vi "Json Parse.vi"(8 "error in (no error)":errorcluster, 11 "JSON":string) -> (0 "error out":errorcluster, 3 "variant":variant)   [LabVIEW 2020, in "WebView2 Control.xctl"]
uses:
  WebView2 Control.xctl
  System.Web.Extensions
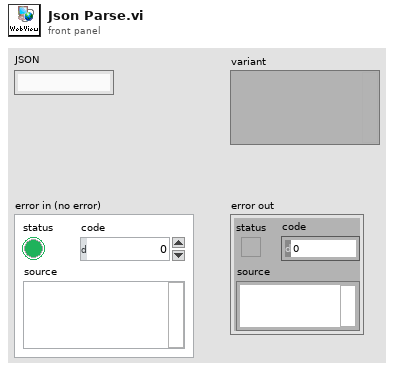
[diagram p1: front panel]
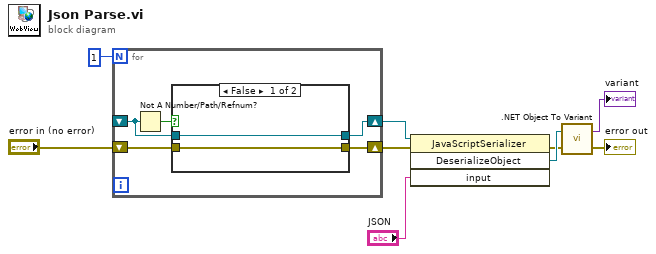
[diagram p0: block diagram]
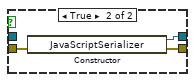
[diagram p2: hidden frame]
diagram:
  n1 = for {
    N: 1 -> [_]
    shift-right: [w14] -> w9
    shift-left: "error in (no error)" -> [w12]
    shift-right: [w13] -> w8
    shift-left: _ -> [w10]
    n2 = Not A Number/Path/Refnum?(number/path/refnum=w10) -> (NaN/Path/Refnum?=w11:bool)
    n3 = case shown="False" w11 {
      tunnel: [w15 w19] -> w14
      tunnel: [w16 w18] -> w13
      tunnel: w12 -> [w15 w17]
      tunnel: w10 -> [w16 _]
      frame False {
      }
      frame True {
        n4 = constructor class="JavaScriptSerializer"(error in=w17) -> (reference out=w18:refnum<k24>, error out=w19:errorcluster)  [unwired: 2 in, 1 out]
      }
    }
  }
  n5 = invoke class="JavaScriptSerializer" method="DeserializeObject"(reference=w8, error in=w9, "input"="JSON") -> (error out=w2:errorcluster, "DeserializeObject"=w6:refnum<k24>)  [unwired: 1 in, 2 out]
  n6 = call <vilib>:".NET Object To Variant.vi"("error in (no error)"=w2, ".NET object"=w6) -> ("error out"=→"error out":errorcluster, "variant"=→"variant":variant)
